vi "parseReportCalibrationDataFrame.vi"(8 "error in (no error)":errorcluster, 10 "ModbusBuffer in":refnum<class "ModbusBuffer.lvclass">, 11 "ILC in":refnum<class "ILC.lvclass">) -> (0 "error out":errorcluster, 2 "ModbusBuffer out":refnum<class "ModbusBuffer.lvclass">, 3 "ILC out":refnum<class "ILC.lvclass">)   [LabVIEW 2016, in "RTILC.lvlib" / "ILC.lvclass"]
uses:
  ILC.lvclass
  Common_RT_Modbus/ModbusBuffer/ModbusBuffer.lvclass
  Common_RT_Modbus/DataTypes/ExceptionCodes.ctl
  Common_RT_Modbus/ModbusBuffer/ModbusBuffer.lvclass/ModbusBuffer.ctl
  ILC.lvclass/ILC.ctl
  Common_RT_Modbus/ModbusBuffer/readInstructionByte.vi
  Common_RT_Modbus/ModbusBuffer/readU8.vi
  Common_RT_Modbus/ModbusBuffer/readTimestampByte.vi
  Common_RT_Modbus/RTModbus.lvlib
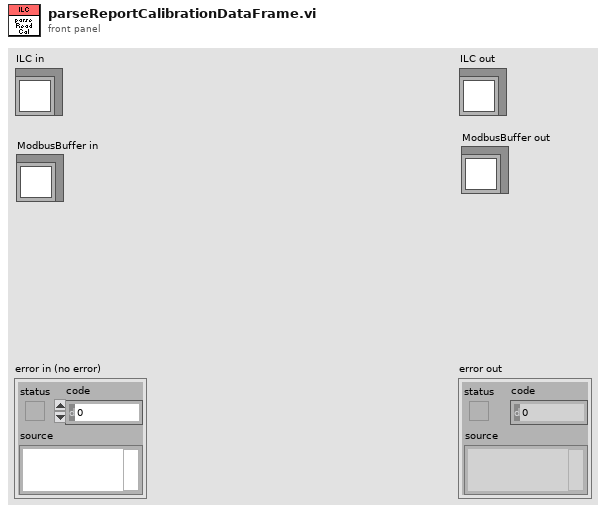
[diagram p1: front panel]
types:
  T1 = typedef "RTModbus.lvlib/ExceptionCodes.ctl" = u16
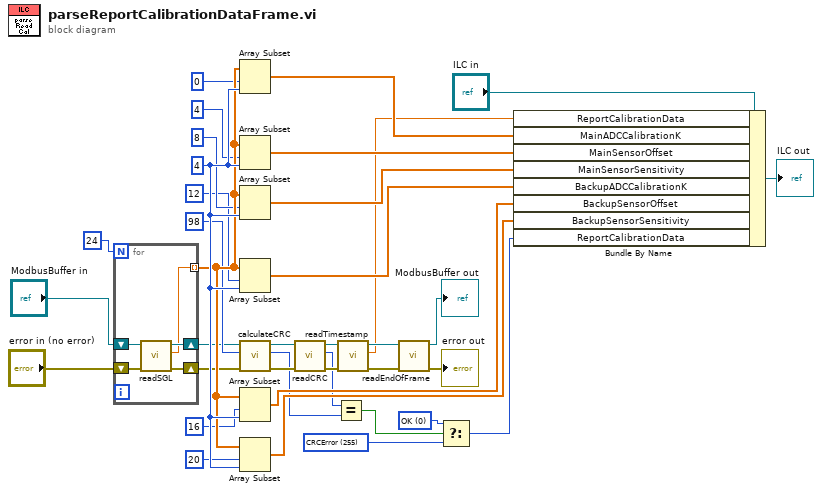
[diagram p0: block diagram]
diagram:
  w18 = T1 255 items=["OK"=0, "IllegalFunction"=1, "IllegalDataAddress"=2, "IllegalDataValue"=3, "SlaveDeviceFailure"=4, "Acknowledge"=5, "SlaveDeviceBusy"=6, "NegativeAcknowledge"=7, "MemoryParityError"=8, "GatewayPathUnavailable"=9, "GatewayTargetDeviceFailedToRespond"=10, "WaitingForResponse"=254, "CRCError"=255] ("f")
  w19 = T1 0 items=["OK"=0, "IllegalFunction"=1, "IllegalDataAddress"=2, "IllegalDataValue"=3, "SlaveDeviceFailure"=4, "Acknowledge"=5, "SlaveDeviceBusy"=6, "NegativeAcknowledge"=7, "MemoryParityError"=8, "GatewayPathUnavailable"=9, "GatewayTargetDeviceFailedToRespond"=10, "WaitingForResponse"=254, "CRCError"=255] ("Responses.ADCOffsetSensitivity")
  w35 = 4
  n1 = for {
    N: 24 -> [_]
    shift-right: [w41] -> w6
    shift-left: "ModbusBuffer in" -> [w42]
    tunnel: [w38] -> w33 mode=indexing
    shift-right: [w40] -> w4
    shift-left: "error in (no error)" -> [w39]
    n2 = call "readSGL.vi"("error in (no error)"=w39, "ModbusBuffer in"=w42) -> ("error out"=w40:errorcluster, "Output"=w38:sgl, "ModbusBuffer out"=w41:refnum<class "ModbusBuffer.lvclass">)  [unwired: 7 in]
  }
  n3 = Array Subset(array=w33, index=0, length=w35) -> (w21:sgl[])
  n4 = Array Subset(array=w33, index=4, length=w35) -> (w22:sgl[])
  n5 = Array Subset(array=w33, index=8, length=w35) -> (w23:sgl[])
  n6 = Array Subset(array=w33, index=12, length=w35) -> (w24:sgl[])
  n7 = call "calculateCRC.vi"("error in (no error)"=w4, "Length"=98, "ModbusBuffer in"=w6) -> ("error out"=w12:errorcluster, "CRC"=w10:u16, "ModbusBuffer out"=w17:refnum<class "ModbusBuffer.lvclass">)  [unwired: 6 in]
  n8 = Array Subset(array=w33, index=16, length=w35) -> (w25:sgl[])
  n9 = Array Subset(array=w33, index=20, length=w35) -> (w26:sgl[])
  n10 = call "readCRC.vi"("error in (no error)"=w12, "ModbusBuffer in"=w17) -> ("error out"=w13:errorcluster, "Output"=w9:u16, "ModbusBuffer out"=w16:refnum<class "ModbusBuffer.lvclass">)  [unwired: 7 in]
  n11 = Equal?(x=w9, y=w10) -> (x = y?=w20:bool)
  n12 = call "readTimestamp.vi"("error in (no error)"=w13, "ModbusBuffer in"=w16) -> ("error out"=w14:errorcluster, "Output"=w7:dbl, "ModbusBuffer out"=w15:refnum<class "ModbusBuffer.lvclass">)  [unwired: 7 in]
  n13 = call "readEndOfFrame.vi"("error in (no error)"=w14, "ModbusBuffer in"=w15) -> ("error out"=→"error out":errorcluster, "ModbusBuffer out"=→"ModbusBuffer out":refnum<class "ModbusBuffer.lvclass">)  [unwired: 8 in]
  n14 = Select(t=w19, s=w20, f=w18) -> (s? t:f=w8:T1)
  n15 = Bundle By Name(cluster="ILC in", "ReportCalibrationData"=w7, "MainADCCalibrationK"=w21, "MainSensorOffset"=w22, "MainSensorSensitivity"=w23, "BackupADCCalibrationK"=w24, "BackupSensorOffset"=w25, "BackupSensorSensitivity"=w26, "ReportCalibrationData"=w8) -> (→"ILC out":refnum<class "ILC.lvclass">)
